vi "2Cnts.vi"(0 "Array Background":dbl[](array[numeric]), 1 "Pow W":dbl, 2 "AcqTime ms":dbl, 3 "Cnts Ref":refnum<vi>, 4 "Display Mode":u16(ring) items=["Sum", "Max", "Sum/s", "Max/s", "Efficiency"], 5 "Array":dbl[](array[numeric])) -> ()   [LabVIEW 2019]
panel:
  out "Value":dbl
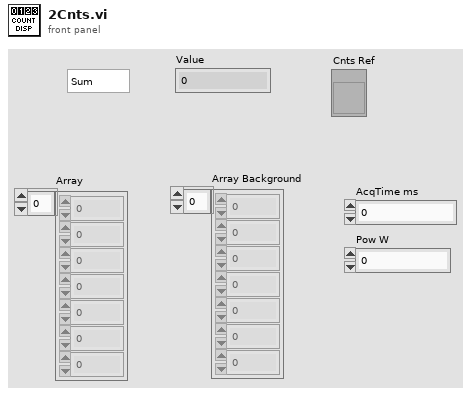
[diagram p1: front panel]
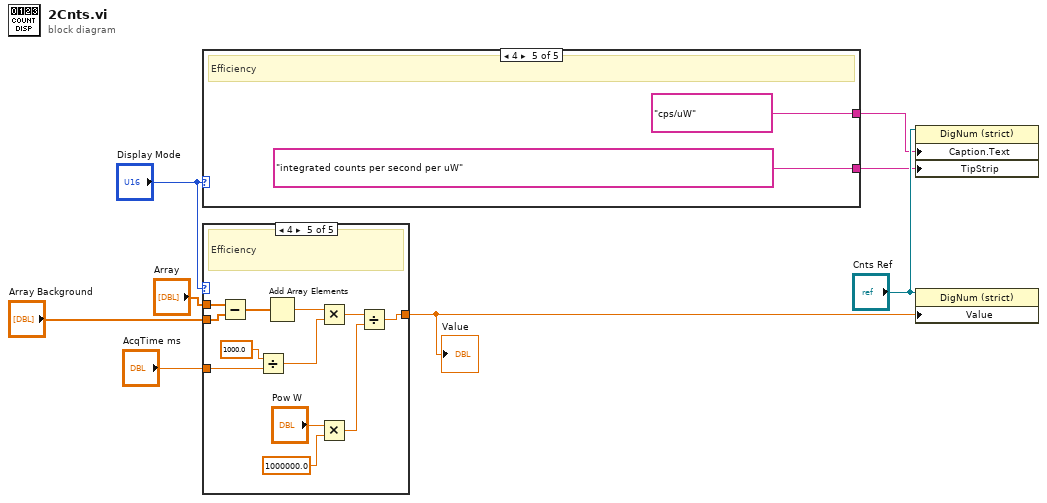
[diagram p0: block diagram]
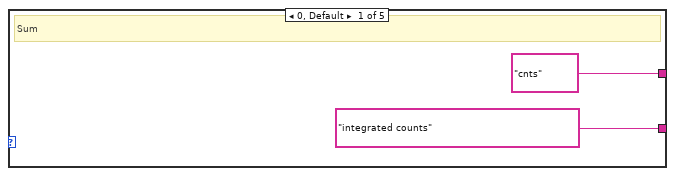
[diagram p2: hidden frame]
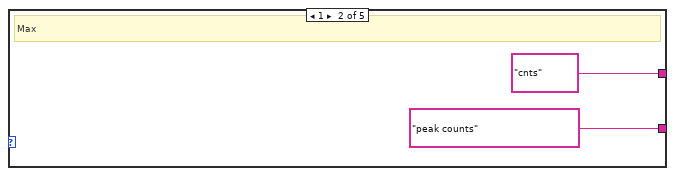
[diagram p3: hidden frame]
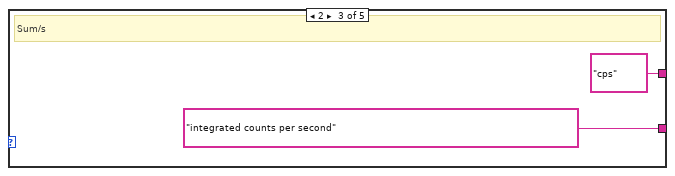
[diagram p4: hidden frame]
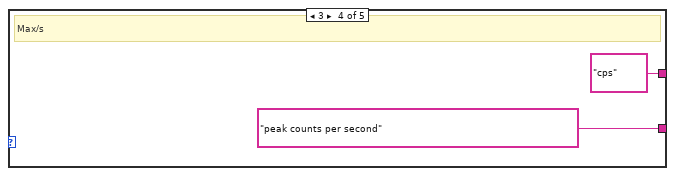
[diagram p5: hidden frame]
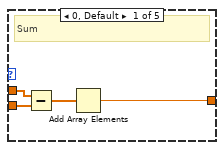
[diagram p6: hidden frame]
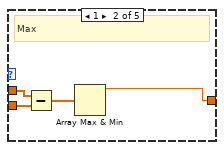
[diagram p7: hidden frame]
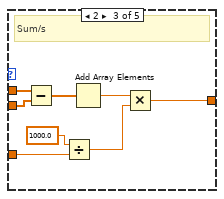
[diagram p8: hidden frame]
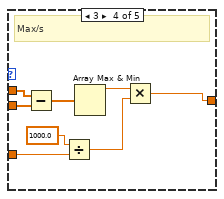
[diagram p9: hidden frame]
diagram:
  n1 = case shown="4" "Display Mode" {
    tunnel: ["cnts" "cnts" "cps" "cps" "cps/uW"] -> w2
    tunnel: ["integrated counts" "peak counts" "integrated counts per second" "peak counts per second" "integrated counts per second per uW"] -> w1
    frame 0, Default {
      # "Sum"
    }
    frame 1 {
      # "Max"
    }
    frame 2 {
      # "Sum/s"
    }
    frame 3 {
      # "Max/s"
    }
    frame 4 {
      # "Efficiency"
    }
  }
  n2 = case shown="4" "Display Mode" {
    tunnel: "AcqTime ms" -> [_ _ w28 w36 w47]
    tunnel: "Array Background" -> [w21 w25 w32 w40 w45]
    tunnel: "Array" -> [w22 w26 w33 w41 w44]
    tunnel: [w19 w23 w27 w35 w43] -> w5
    frame 0, Default {
      # "Sum"
      n3 = Subtract(x=w22, y=w21) -> (x-y=w20:dbl[])
      n4 = Add Array Elements(numeric array=w20) -> (sum=w19:dbl)
    }
    frame 1 {
      # "Max"
      n5 = Subtract(x=w26, y=w25) -> (x-y=w24:dbl[])
      n6 = Array Max & Min(array=w24) -> (max value=w23:dbl)  [unwired: 3 out]
    }
    frame 2 {
      # "Sum/s"
      n7 = Subtract(x=w33, y=w32) -> (x-y=w34:dbl[])
      n8 = Divide(x=1000.0, y=w28) -> (x/y=w31:dbl)
      n9 = Add Array Elements(numeric array=w34) -> (sum=w29:dbl)
      n10 = Multiply(x=w29, y=w31) -> (x*y=w27:dbl)
    }
    frame 3 {
      # "Max/s"
      n11 = Subtract(x=w41, y=w40) -> (x-y=w42:dbl[])
      n12 = Divide(x=1000.0, y=w36) -> (x/y=w39:dbl)
      n13 = Array Max & Min(array=w42) -> (max value=w37:dbl)  [unwired: 3 out]
      n14 = Multiply(x=w37, y=w39) -> (x*y=w35:dbl)
    }
    frame 4 {
      # "Efficiency"
      n15 = Subtract(x=w44, y=w45) -> (x-y=w51:dbl[])
      n16 = Divide(x=1000.0, y=w47) -> (x/y=w49:dbl)
      n17 = Add Array Elements(numeric array=w51) -> (sum=w52:dbl)
      n18 = Multiply(x=w52, y=w49) -> (x*y=w50:dbl)
      n19 = Multiply(x="Pow W", y=1000000.0) -> (x*y=w48:dbl)
      n20 = Divide(x=w50, y=w48) -> (x/y=w43:dbl)
    }
  }
  "Value" <- w5
  n21 = property class="DigNum (strict)"(reference="Cnts Ref", "Caption.Text"=w2, "TipStrip"=w1) -> ()  [unwired: 1 in, 2 out]
  n22 = property class="DigNum (strict)"(reference="Cnts Ref", "Value"=w5) -> ()  [unwired: 1 in, 2 out]
